vi "Robot Main.vi"() -> ()   [LabVIEW 2016]
doc: "This VI implements the framework and scheduler for your robotics program. It should not be necessary to modify the framework. You are expected to add your code to the VIs called from Robot Main - the ones located in the Team Code folder within the project."
uses:
  Robot Global Data.vi
  <vilib>/Rock Robotics/WPI/Camera/WPI_CameraImageSize.ctl
panel:
  in  "Finish 3":bool
  in  "Enable Vision 3":bool
  in  "Image Size 3":T1=enum."320x240"
  in  "Code Writer":enum16{"Cheeto", "Ian", "Curtis"}(ring)
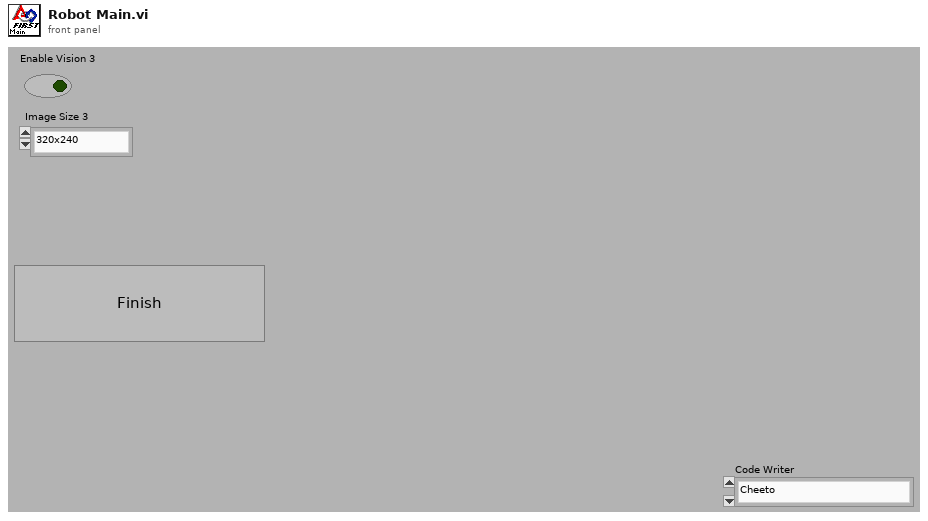
[diagram p1: front panel]
types:
  T1 = typedef "WPI_CameraImageSize.ctl" = enum16{"640x480", "320x240", "160x120", "Custom"}
  T2 = typedef "WPI_DriverStationMatch Info.ctl" = cluster{"Autonomous Elapsed Seconds":dbl, "TeleOp Elapsed Seconds":dbl, "Disabled Elapsed Seconds":dbl, "Visited Autonomous":bool, "Visited TeleOp":bool, "Visited Disabled":bool, "Autonomous Settings":cluster{"Autonomous Style":enum16{"Iterative", "Independent"}, "VI Refnum":refnum<vi>}}
  T3 = typedef "WPI_DriverStationDerivedRobotMode.ctl" = enum16{"Init", "Execute", "Stop"}
  T4 = typedef "WPI_DriverStationRobotMode2.ctl" = enum16{"Autonomous Disabled", "Autonomous Enabled", "Teleop Disabled", "Teleop Enabled", "Disconnected", "Finish", "Test Disabled", "Test Enabled", "Emergency Stopped"}
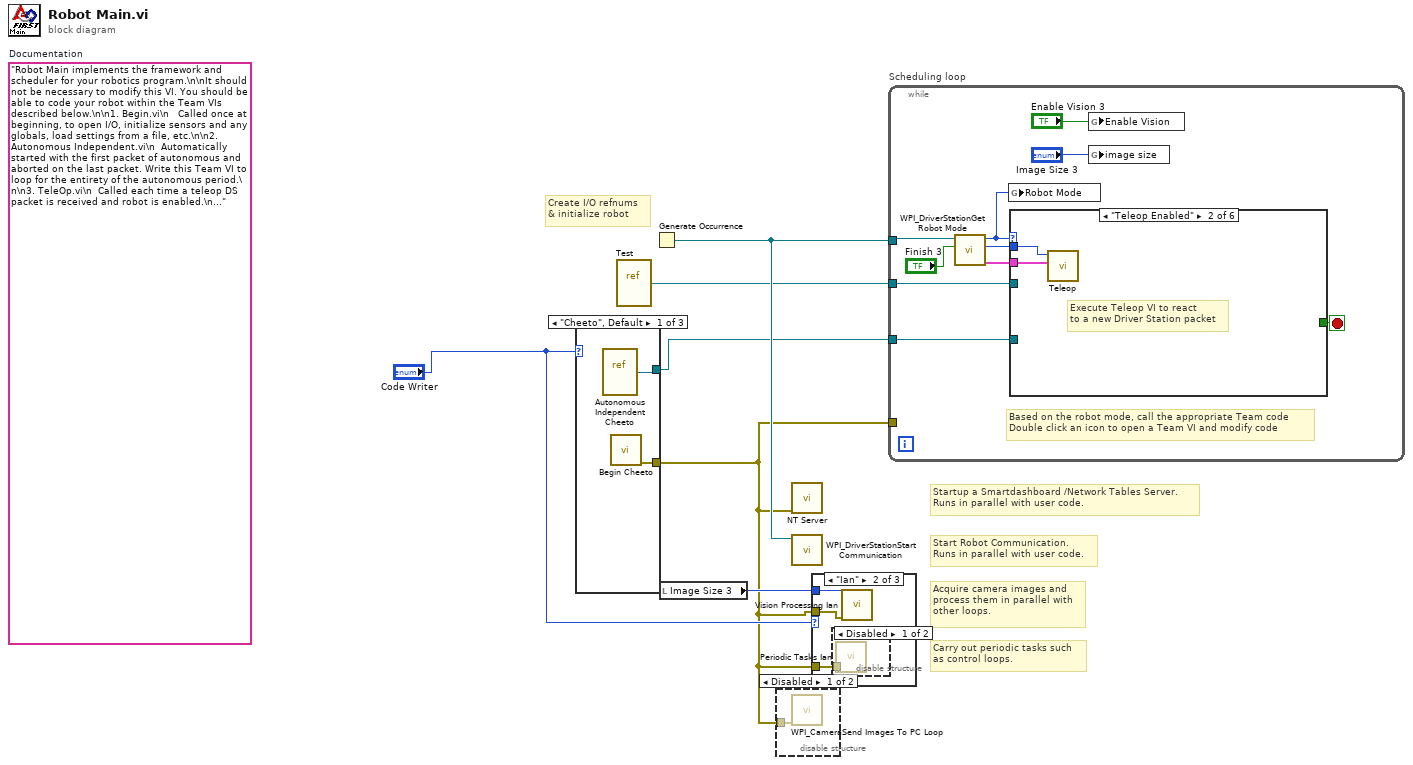
[diagram p0: block diagram]
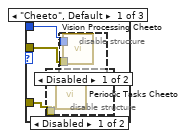
[diagram p3: hidden frame]
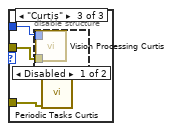
[diagram p7: hidden frame]
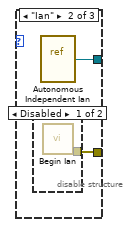
[diagram p9: hidden frame]
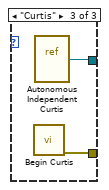
[diagram p11: hidden frame]
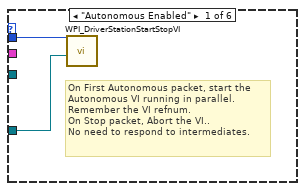
[diagram p12: hidden frame]
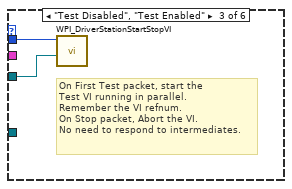
[diagram p13: hidden frame]
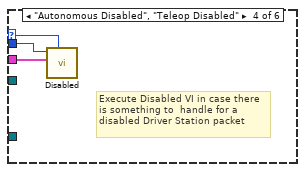
[diagram p14: hidden frame]
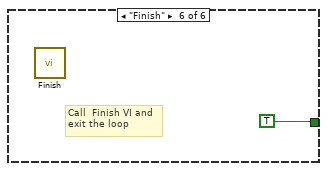
[diagram p16: hidden frame]
diagram:
  (unwired) "Robot Main implements the framework and scheduler for your robotics program.\n\nIt should not be necessary to modify this VI. You should be able to code your robot within the Team VIs described below.\n\n1. Begin.vi\n   Called once at beginning, to open I/O, initialize sensors and any globals, load settings from a file, etc.\n\n2. Autonomous Independent.vi\n  Automatically started with the first packet of autonomous and aborted on the last packet. Write this Team VI to loop for the entirety of the autonomous period.\n\n3. TeleOp.vi\n  Called each time a teleop DS packet is received and robot is enabled.\n\n4. Disabled.vi\n  Called each time a packet is received and the robot is disabled.\n\n5. Test.vi\n  Called Automatically started with the first test packet and aborted on the last. Modify this VI to carry out robot and sensor validation tests.\n\n6. Vision.vi\n  A parallel loop that acquires and processes camera images.\n\n7. PeriodicTasks.vi\n  Parallel loops running at user-defined rates.\n\n8. Finish.vi\n  Called before exiting, so you can save data, clean up I/O, etc.\n"  # Documentation
  # "Startup a Smartdashboard /Network Tables Server.\nRuns in parallel with user code."
  # "Carry out periodic tasks such\nas control loops."
  # "Acquire camera images and\nprocess them in parallel with\nother loops."
  # "Create I/O refnums\n& initialize robot"
  # "Start Robot Communication.\nRuns in parallel with user code."
  n1 = case shown="\"Cheeto\", Default" "Code Writer" {
    tunnel: [w8 w10 w13] -> w4
    tunnel: [w7 w9 w12] -> w1
    frame "Cheeto", Default {
      n2 = vi-ref "Autonomous Independent Cheeto.vi"() -> (w8:refnum<vi>)
      n3 = call "Begin Cheeto.vi"() -> ("error out"=w7:errorcluster)  [unwired: 11 in]
    }
    frame "Ian" {
      n4 = disable-structure shown="Disabled" {
        disable-tunnel: [w11 _] -> w9
        frame Disabled {
          n5 = call "Begin Ian.vi"() -> ("error out"=w11:errorcluster)  [unwired: 11 in]
        }
        frame Enabled {
        }
      }
      n6 = vi-ref "Autonomous Independent Ian.vi"() -> (w10:refnum<vi>)
    }
    frame "Curtis" {
      n7 = call "Begin Curtis.vi"() -> ("error out"=w12:errorcluster)  [unwired: 11 in]
      n8 = vi-ref "Autonomous Independent Curtis.vi"() -> (w13:refnum<vi>)
    }
  }
  n9 = vi-ref "Test.vi"() -> (w5:refnum<vi>)
  n10 = Generate Occurrence() -> (w6:refnum<k4>)
  n11 = local read "Image Size 3"() -> (w2:T1)
  n12 = disable-structure shown="Disabled" {
    disable-tunnel: w1 -> [w14 _]
    frame Disabled {
      n13 = call <vilib>:"WPI_CameraSend Images To PC Loop.vi"("error in (no error)"=w14) -> ()  [unwired: 11 in]
    }
    frame Enabled {
    }
  }
  n14 = call <vilib>:"NT Server.vi"("error in (no error)"=w1) -> ()  [unwired: 11 in]
  n15 = call <vilib>:"WPI_DriverStationStart Communication.vi"("occurrence"=w6) -> ()  [unwired: 1 in, 10 out]
  n16 = case shown="\"Ian\"" "Code Writer" {
    tunnel: w1 -> [w17 w23 w27]
    tunnel: w2 -> [w16 w21 w26]
    tunnel: w1 -> [w15 w22 w25]
    frame "Cheeto", Default {
      n17 = disable-structure shown="Disabled" {
        disable-tunnel: w17 -> [w18 _]
        frame Disabled {
          n18 = call "Periodic Tasks Cheeto.vi"("error in"=w18) -> ()  [unwired: 11 in]
        }
        frame Enabled {
        }
      }
      n19 = disable-structure shown="Disabled" {
        disable-tunnel: w16 -> [w20 _]
        disable-tunnel: w15 -> [w19 _]
        frame Disabled {
          n20 = call "Vision Processing Cheeto.vi"("error in (no error)"=w19, "Image Size"=w20) -> ()  [unwired: 6 in]
        }
        frame Enabled {
        }
      }
    }
    frame "Ian" {
      n21 = disable-structure shown="Disabled" {
        disable-tunnel: w23 -> [w24 _]
        frame Disabled {
          n22 = call "Periodic Tasks Ian.vi"("error in"=w24) -> ()  [unwired: 11 in]
        }
        frame Enabled {
        }
      }
      n23 = call "Vision Processing Ian.vi"("error in (no error)"=w22, "Image Size Gear"=w21) -> ()  [unwired: 6 in]
    }
    frame "Curtis" {
      n24 = disable-structure shown="Disabled" {
        disable-tunnel: w26 -> [w29 _]
        disable-tunnel: w25 -> [w28 _]
        frame Disabled {
          n25 = call "Vision Processing Curtis.vi"("error in (no error)"=w28, "Image Size"=w29) -> ()  [unwired: 6 in]
        }
        frame Enabled {
        }
      }
      n26 = call "Periodic Tasks Curtis.vi"("error in"=w27) -> ()  [unwired: 11 in]
    }
  }
  n27 = while "Scheduling loop" {
    tunnel: w6 -> [w38]
    tunnel: w1 -> [_]
    tunnel: w4 -> [w33]
    tunnel: w5 -> [w31]
    stop <- w35 stop-if-true
    # "Based on the robot mode, call the appropriate Team code\nDouble click an icon to open a Team VI and modify code"
    n28 = call <vilib>:"WPI_DriverStationGet Robot Mode.vi"("Finish"="Finish 3", "DS Occurrence"=w38) -> ("Match Info out"=w36:T2, "Call Context"=w39:T3, "Robot Mode"=w30:T4)  [unwired: 7 out]
    n29 = global write "Robot Global Data.vi" "Robot Mode"(w30) -> ()
    n30 = case shown="\"Teleop Enabled\"" w30 {
      selector: w30 -> [_ _ _ w46 _ _]
      tunnel: w39 -> [w41 w43 w45 w48 _ _]
      tunnel: w36 -> [_ w42 _ w47 _ _]
      tunnel: [_ _ _ _ _ TRUE] -> w35
      tunnel: w33 -> [w40 _ _ _ _ _]
      tunnel: w31 -> [_ _ w44 _ _ _]
      frame "Autonomous Enabled" {
        # "On First Autonomous packet, start the\nAutonomous VI running in parallel.\nRemember the VI refnum.\nOn Stop packet, Abort the VI..\nNo need to respond to intermediates."
        n31 = call <vilib>:"WPI_DriverStationStartStopVI.vi"("VI in"=w40, "Call Context"=w41) -> ()  [unwired: 10 in]
      }
      frame "Teleop Enabled" {
        # "Execute Teleop VI to react\nto a new Driver Station packet"
        n32 = call "Teleop.vi"("Match Info"=w42, "Call Context"=w43) -> ()  [unwired: 1 in, 9 out]
      }
      frame "Test Disabled", "Test Enabled" {
        # "On First Test packet, start the\nTest VI running in parallel.\nRemember the VI refnum.\nOn Stop packet, Abort the VI.\nNo need to respond to intermediates."
        n33 = call <vilib>:"WPI_DriverStationStartStopVI.vi"("VI in"=w44, "Call Context"=w45) -> ()  [unwired: 10 in]
      }
      frame "Autonomous Disabled", "Teleop Disabled" {
        # "Execute Disabled VI in case there\nis something to  handle for a\ndisabled Driver Station packet"
        n34 = call "Disabled.vi"("Robot Mode"=w46, "Match Info"=w47, "Call Context"=w48) -> ()  [unwired: 1 in, 8 out]
      }
      frame "Disconnected", Default {
        # "Driver Station packet didn't arrive.\nPossibly useful for diagnostics"
      }
      frame "Finish" {
        # "Call  Finish VI and\nexit the loop"
        n35 = call "Finish.vi"() -> ()  [unwired: 1 in, 7 out]
      }
    }
    n36 = global write "Robot Global Data.vi" "Enable Vision"("Enable Vision 3") -> ()
    n37 = global write "Robot Global Data.vi" "image size"("Image Size 3") -> ()
  }
